vi "Configure List Step Value.vi"(7 "Step Type":u16(ring) items=["Voltage", "Current", "Slew", "Width"], 8 "error in":errorcluster, 9 "Value":dbl min=0.0, 10 "List Step":u8=1 min=1 max=100 step=1, 11 "VISA resource name":refnum<visa-resource-name>) -> (0 "error out":errorcluster, 3 "VISA resource name out":refnum<visa-resource-name>)   [LabVIEW 2018, in "IT-M3100.lvlib"]
doc: "This command to set the list of single step value.\n<b>Step Type</b>\n0:Voltage:This command sets the voltage value of the nth step in the list program.\n1:Current:This command sets the current value of the nth step in the list program.\n2:Slew:This command sets the slew rate value of the nth step in the list program.\n3:Width:This command sets the width value of the nth step in the list program.\n<b>List Step</b>\n1-100\n<b>Value</b>\n0-MAX"
uses:
  IT-M3100.lvlib
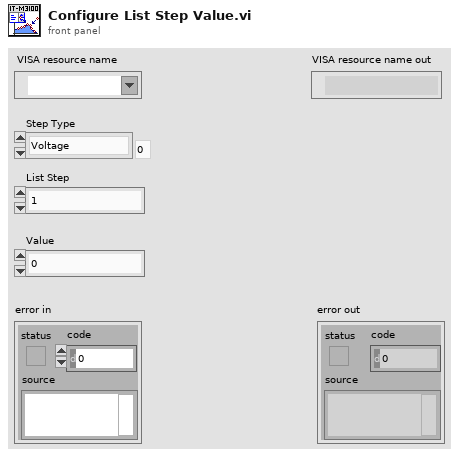
[diagram p1: front panel]
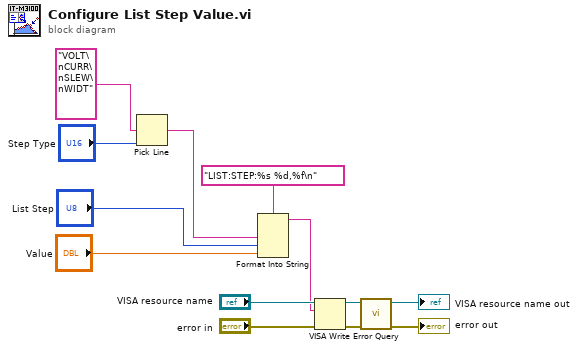
[diagram p0: block diagram]
diagram:
  n1 = Pick Line(multi-line string="VOLT\nCURR\nSLEW\nWIDT", line index="Step Type") -> (output string=w3:string)  [unwired: 1 in]
  n2 = Format Into String(format string="LIST:STEP:%s %d,%f\n", w3, "List Step", "Value") -> (resulting string=w6:string)  [unwired: 2 in, 1 out]
  n3 = VISA Write(VISA resource name="VISA resource name", write buffer=w6, error in (no error)="error in") -> (VISA resource name out=w10:refnum<visa-resource-name>, error out=w11:errorcluster)  [unwired: 1 out]
  n4 = call "Error Query.vi"("error in"=w11, "VISA resource name"=w10) -> ("error out"=→"error out":errorcluster, "VISA resource name out"=→"VISA resource name out":refnum<visa-resource-name>)  [unwired: 6 in, 2 out]
